vi "capstone1 ver 6.vi"() -> ()   [LabVIEW 2016]
uses:
  <instrlib>/Dynamixel Motor/Public/Motor Operation/Low Level/Baud Setting.ctl
  <vilib>/myRIO/Instrument Drivers/Onboard IO/DIO/typedefs/DIO Reference.ctl
  <vilib>/myRIO/Common/Instrument Driver Framework/Utilities/typedefs/myRIO Generic Hardware Reference.ctl
  <vilib>/myRIO/Common/Instrument Driver Framework/Utilities/typedefs/Hardware Version Enum.ctl
  <vilib>/myRIO/Common/Instrument Driver Framework/Utilities/typedefs/myRIO v1.0 Reference.ctl
  <vilib>/myRIO/Common/Instrument Driver Framework/Utilities/typedefs/Generic FPGA Reference.ctl
  <vilib>/myRIO/Common/Instrument Driver Framework/myRIO v1.0/DIO/typedefs/DIO Channels List.ctl
  <vilib>/myRIO/Common/Instrument Driver Framework/myRIO v1.0/DIO/typedefs/DIO Channels Enum.ctl
  <vilib>/userdefined/High Color/nirio_resource_hc.ctl
  <vilib>/myRIO/Instrument Drivers/Onboard IO/AI/typedefs/AI Reference.ctl
  <vilib>/myRIO/Common/Instrument Driver Framework/myRIO v1.0/AI/typedefs/AI Channels List.ctl
  <vilib>/myRIO/Common/Instrument Driver Framework/myRIO v1.0/AI/typedefs/AI Channels Enum.ctl
  <vilib>/myRIO/Common/Instrument Driver Framework/Utilities/typedefs/Analog Scaling Constants List.ctl
  <vilib>/myRIO/Common/Instrument Driver Framework/Utilities/typedefs/Analog Scaling Constants.ctl
  <vilib>/myRIO/Instrument Drivers/Onboard IO/AO/typedefs/AO Reference.ctl
  <vilib>/myRIO/Common/Instrument Driver Framework/myRIO v1.0/AO/typedefs/AO Channels List.ctl
  <vilib>/myRIO/Common/Instrument Driver Framework/myRIO v1.0/AO/typedefs/AO Channels Enum.ctl
  <vilib>/myRIO/Common/Instrument Driver Framework/Utilities/vis/Is FPGA Ref Available.vi
  <vilib>/myRIO/Common/Instrument Driver Framework/myRIO v1.0/DIO/vis/myRIO v1.1 Open DIO.vi
  <vilib>/myRIO/Instrument Drivers/Onboard IO/DIO/vis/Write.vi
  <vilib>/myRIO/Common/Instrument Driver Framework/myRIO v1.0/AI/vis/myRIO v1.1 Open AI.vi
  <vilib>/myRIO/Instrument Drivers/Onboard IO/AI/vis/Read.vi
  <vilib>/myRIO/Common/Instrument Driver Framework/myRIO v1.0/AO/vis/myRIO v1.1 Open AO.vi
  <vilib>/myRIO/Instrument Drivers/Onboard IO/AO/vis/Write.vi
  <vilib>/myRIO/Common/Instrument Driver Framework/Utilities/vis/Validate Channels.vi
  <vilib>/myRIO/Common/Instrument Driver Framework/myRIO v1.0/DIO/vis/myRIO v1.0 Reserve DIO.vi
  <vilib>/myRIO/Common/Instrument Driver Framework/myRIO v1.0/AI/vis/myRIO v1.0 Reserve AI.vi
  <vilib>/myRIO/Common/Instrument Driver Framework/myRIO v1.0/AO/vis/myRIO v1.0 Reserve AO.vi
  <vilib>/myRIO/Common/Instrument Driver Framework/myRIO v1.0/UART/vis/myRIO v1.0 Close UART.vi
  <vilib>/myRIO/Common/Instrument Driver Framework/myRIO v1.0/Resource Manager/vis/myRIO v1.0 Reserve Channel List.vi
  <vilib>/myRIO/Common/Instrument Driver Framework/myRIO v1.0/DIO/vis/myRIO v1.0 Build MUX Configuration DIO.vi
  <vilib>/myRIO/Common/Instrument Driver Framework/myRIO v1.0/AI/vis/myRIO v1.0 Build MUX Configuration AI.vi
  <vilib>/myRIO/Common/Instrument Driver Framework/myRIO v1.0/AO/vis/myRIO v1.0 Build MUX Configuration AO.vi
  <vilib>/myRIO/Common/Instrument Driver Framework/myRIO v1.0/Resource Manager/vis/myRIO v1.0 Reserve Channel.vi
  <vilib>/myRIO/Common/Instrument Driver Framework/myRIO v1.0/Resource Manager/vis/myRIO v1.0 Unreserve Channel.vi
  <vilib>/myRIO/Common/Instrument Driver Framework/myRIO v1.0/Resource Manager/vis/myRIO v1.0 Create Configuration List.vi
  <vilib>/myRIO/Common/Instrument Driver Framework/myRIO v1.0/Resource Manager/vis/myRIO v1.0 Build Mutex Name.vi
  <vilib>/Utility/VariantDataType/GetNumericInfo.vi
  <vilib>/Utility/error.llb/Error Cluster From Error Code.vi
  <vilib>/myRIO/Common/Instrument Driver Framework/myRIO v1.0/myRIO v1.1 Open.vi
  <vilib>/myRIO/Common/Instrument Driver Framework/Utilities/vis/IO Manager.vi
  <vilib>/myRIO/Common/Instrument Driver Framework/Utilities/vis/Configuration Manager.vi
  <vilib>/myRIO/Common/Instrument Driver Framework/myRIO v1.0/Resource Manager/vis/myRIO v1.0 Configure IO.vi
  <vilib>/myRIO/Common/Instrument Driver Framework/myRIO v1.0/myRIO v1.0 Close.vi
  <vilib>/myRIO/Common/Instrument Driver Framework/myRIO v1.0/DIO/vis/myRIO v1.0 Write DIO.vi
  <vilib>/myRIO/Common/Instrument Driver Framework/myRIO v1.0/AI/vis/myRIO v1.0 Get Scaling Constants AI.vi
  <vilib>/myRIO/Common/Instrument Driver Framework/myRIO v1.0/AI/vis/myRIO v1.0 Read AI.vi
  <vilib>/myRIO/Common/Instrument Driver Framework/myRIO v1.0/AO/vis/myRIO v1.0 Get Scaling Constants AO.vi
  <vilib>/myRIO/Common/Instrument Driver Framework/myRIO v1.0/AO/vis/myRIO v1.0 Write AO.vi
  <vilib>/myRIO/Common/Instrument Driver Framework/Utilities/vis/FPGA Ref Manager.vi
  <vilib>/myRIO/Common/Instrument Driver Framework/myRIO v1.0/myRIO v1.0 Reset FPGA.vi
  <vilib>/myRIO/Common/Instrument Driver Framework/myRIO v1.0/IRQ/vis/myRIO v1.0 IRQ Info FGV.vi
  <vilib>/myRIO/Common/Instrument Driver Framework/myRIO v1.0/IRQ/vis/myRIO v1.0 Timer IRQ Info FGV.vi
  <vilib>/myRIO/Common/Instrument Driver Framework/myRIO v1.0/IRQ/vis/myRIO v1.0 ISR Agent.vi
  <vilib>/myRIO/Express VI/Onboard Devices/LED/LED Express VI.xnode
  <vilib>/myRIO/Instrument Drivers/Onboard IO/DIO/vis/myRIO DIO Open.xnode
  <vilib>/myRIO/Express VI/Onboard IO/AI/AI Express VI.xnode
  <vilib>/myRIO/Instrument Drivers/Onboard IO/AI/vis/myRIO AI Open.xnode
  <vilib>/myRIO/Express VI/Onboard IO/AO/AO Express VI.xnode
  <vilib>/myRIO/Instrument Drivers/Onboard IO/AO/vis/myRIO AO Open.xnode
  <instrlib>/Dynamixel Motor/Dynamixel Motor.lvlib
  <vilib>/myRIO/Instrument Drivers/Onboard IO/DIO/DIO.lvlib
  <vilib>/myRIO/Instrument Drivers/Utilities/Utilities.lvlib
  <vilib>/myRIO/Instrument Drivers/Onboard IO/AO/AO.lvlib
  <vilib>/myRIO/Instrument Drivers/Onboard IO/AI/AI.lvlib
panel:
  out "Load/torque % 3":sgl
  out "Load/torque % 2":sgl
  out "Load/torque %":sgl
  in  "main stop":bool
  out "RT TCP Loop time":u32
  out "motor temp":cluster{"0":sgl, "1":sgl, "2":sgl, "3":sgl}
  out "value":T1
  out "TCP Read data":string
  in  "정지":bool
  out "error out":errorcluster
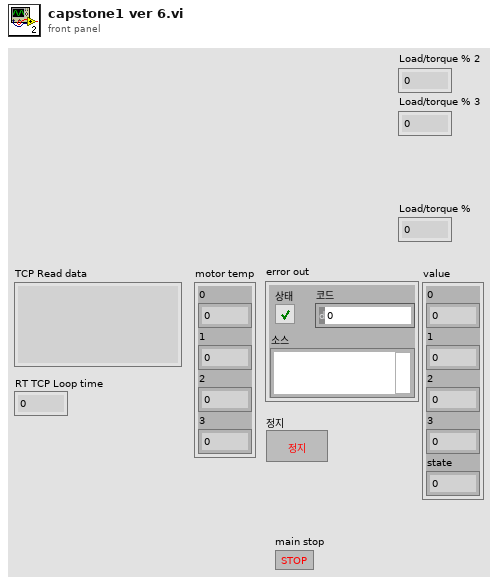
[diagram p1: front panel]
types:
  T1 = cluster{"0":sgl, "1":sgl, "2":sgl, "3":sgl, "state":sgl}
  T2 = typedef "DIO.lvlib/DIO Reference.ctl" = cluster{"myRIO Reference":T3, "DIO Channels List":T7}
  T3 = typedef "myRIO Generic Hardware Reference.ctl" = cluster{"myRIO Model":T4, "myRIO Hardware Reference":T5}
  T4 = typedef "Hardware Version Enum.ctl" = enum16{"Unknown", "myRIO-1900", "myRIO-1950", "roboRIO", "NI ELVIS RIO CM"}
  T5 = typedef "myRIO v1.0 Reference.ctl" = cluster{"Generic FPGA Reference":T6, "Allow multiple opens":bool}
  T6 = typedef "Generic FPGA Reference.ctl" = refnum<k20>
  T7 = typedef "DIO Channels List.ctl" = T8[]
  T8 = typedef "DIO Channels Enum.ctl" = enum16{"Not Connected", "C/DIO0", "C/DIO1", "C/DIO2", "C/DIO3", "C/DIO4", "C/DIO5", "C/DIO6", "C/DIO7", "A/DIO0", "A/DIO1", "A/DIO2", "A/DIO3", "A/DIO4", "A/DIO5", "A/DIO6", "A/DIO7", "A/DIO8", "A/DIO9", "A/DIO10", "A/DIO11", "A/DIO12", "A/DIO13", "A/DIO14", "A/DIO15", "B/DIO0", "B/DIO1", "B/DIO2", "B/DIO3", "B/DIO4", "B/DIO5", "B/DIO6", "B/DIO7", "B/DIO8", "B/DIO9", "B/DIO10", "B/DIO11", "B/DIO12", "B/DIO13", "B/DIO14", "B/DIO15", "LED0", "LED1", "LED2", "LED3", "Button0", "DIO/DIO0", "DIO/DIO1", "DIO/DIO2", "DIO/DIO3", "DIO/DIO4", "DIO/DIO5", "DIO/DIO6", "DIO/DIO7", "DIO/DIO8", "DIO/DIO9", "SPI/CS0", "SPI/CS1", "SPI/CS2", "SPI/CS3", "LED RADIO (Green)", "LED RADIO (Red)", "LED COMM (Green)", "LED COMM (Red)", "LED MODE (Green)", "LED MODE (Red)"}
  T9 = typedef "nirio_resource_hc.ctl" = tag
  T10 = cluster{"0":sgl, "1":sgl, "2":sgl, "3":sgl, "state":i32}
  T11 = typedef "AI.lvlib/AI Reference.ctl" = cluster{"myRIO Reference":T3, "AI Channels List":T12, "AI Scaling Constants List":T14}
  T12 = typedef "AI Channels List.ctl" = T13[]
  T13 = typedef "AI Channels Enum.ctl" = enum16{"Not Connected", "AudioIn/Left", "AudioIn/Right", "C/AI0", "C/AI1", "A/AI0", "A/AI1", "A/AI2", "A/AI3", "B/AI0", "B/AI1", "B/AI2", "B/AI3", "AI/AI0", "AI/AI1", "AI/AI2", "AI/AI3"}
  T14 = typedef "Analog Scaling Constants List.ctl" = T15[]
  T15 = typedef "Analog Scaling Constants.ctl" = cluster{"LSB Weight (Volts)":dbl, "Offset (Volts)":dbl, "Signed?":bool}
  T16 = typedef "AO.lvlib/AO Reference.ctl" = cluster{"myRIO Reference":T3, "AO Channel List":T17, "AO Scaling Constant List":T14}
  T17 = typedef "AO Channels List.ctl" = T18[]
  T18 = typedef "AO Channels Enum.ctl" = enum16{"Not Connected", "AudioOut/Left", "AudioOut/Right", "C/AO0", "C/AO1", "A/AO0", "A/AO1", "B/AO0", "B/AO1"}
  T19 = enum16{"big-endian, network order", "native, host order", "little-endian"}
  T20 = typedef "Dynamixel Motor.lvlib/Baud Setting.ctl" = u8
  T21 = cluster{"Temperature (C)":u8, "Temperature (C)":u8, "Temperature (C)":u8, "Temperature (C)":u8}
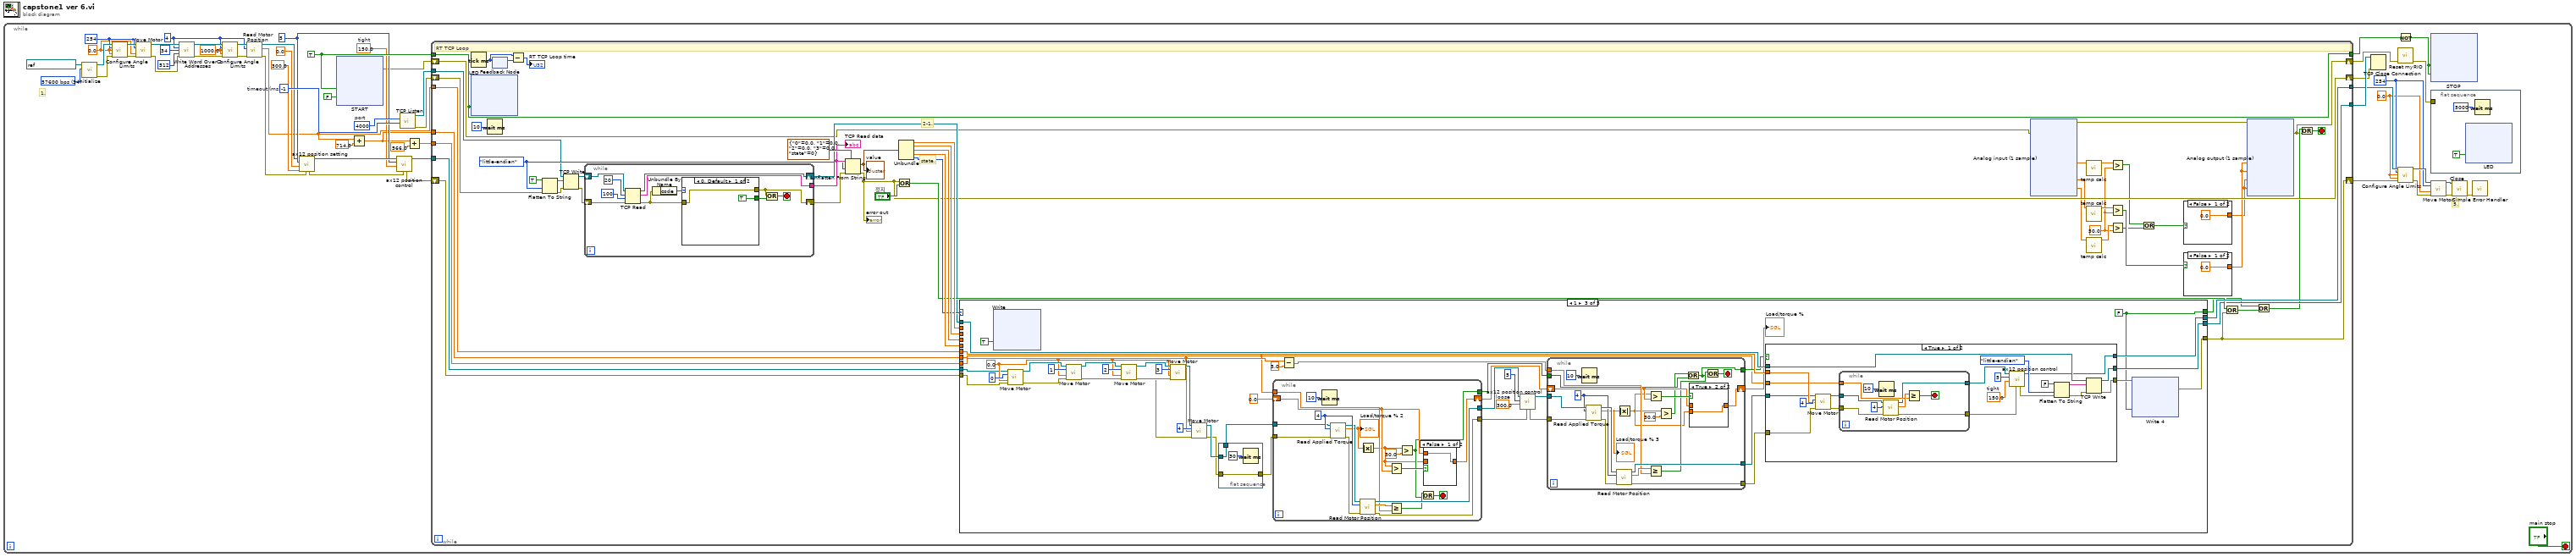
[diagram p0: block diagram]
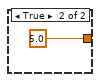
[diagram p2: hidden frame]
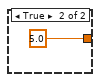
[diagram p3: hidden frame]
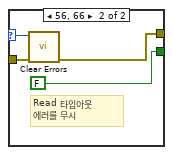
[diagram p4: hidden frame]
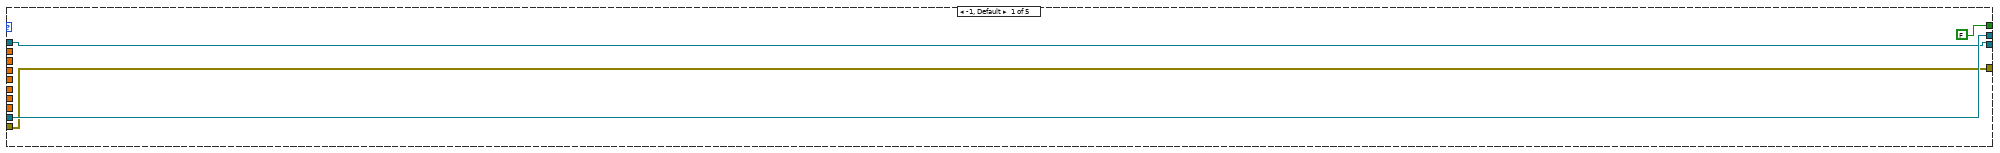
[diagram p5: hidden frame]
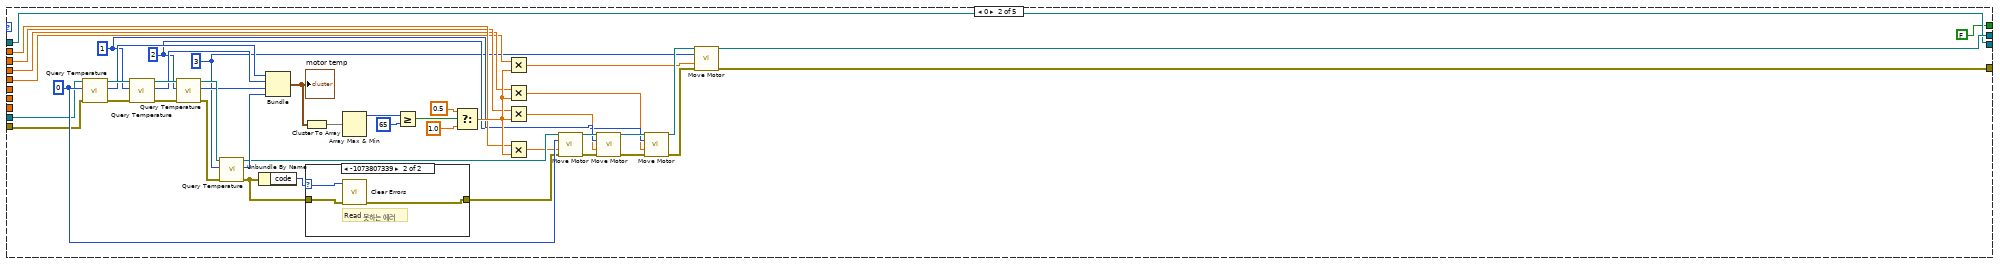
[diagram p6: hidden frame]
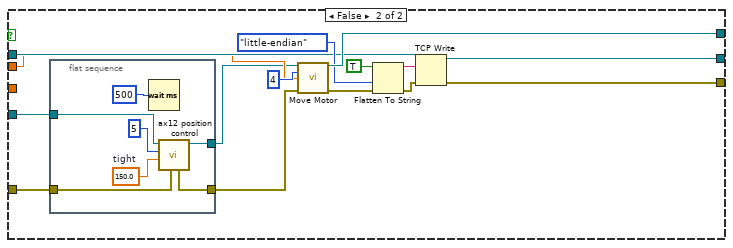
[diagram p8: hidden frame]
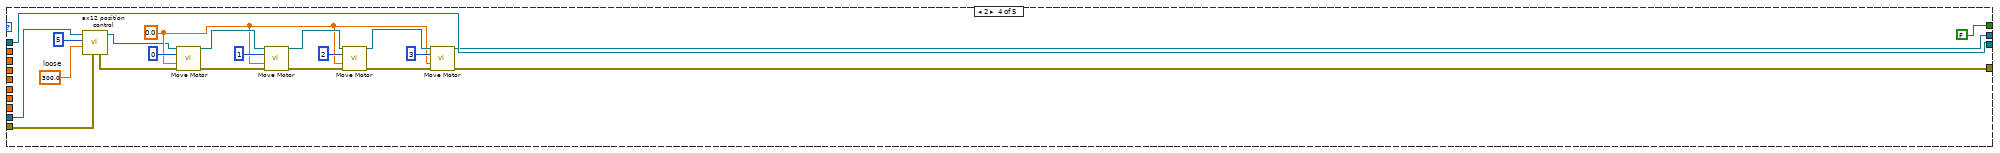
[diagram p11: hidden frame]
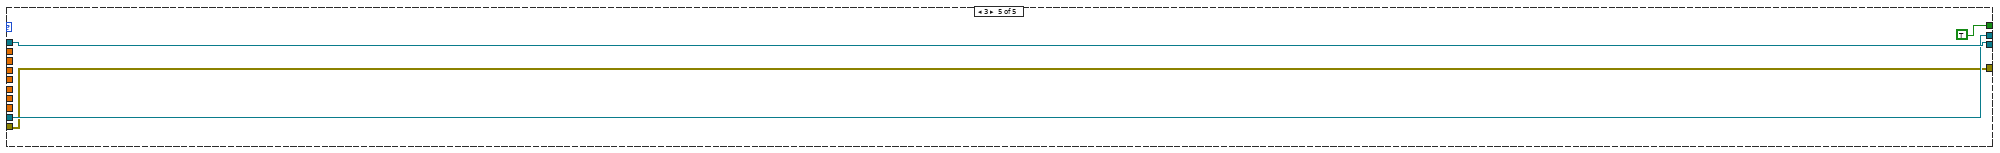
[diagram p12: hidden frame]
diagram:
  n1 = while {
    stop <- "main stop" stop-if-true
    w36 = 1000.0 ("Clockwise Angle Limit (0 deg)")
    w1 = 4
    w29 = 150.0  # tight
    w28 = 5
    w51 = T20 34 items=["1,000,000 bps"=1, "500,000 bps"=3, "400,000 bps"=4, "250,000 bps"=7, "200,000 bps"=9, "115200 bps"=16, "57600 bps"=34, "19200 bps"=103, "9600 bps"=207] ("Baud rate (57600 bps)")
    w41 = TRUE
    w22 = 0.0 ("Goal Speed (RPM)")
    w23 = u8 254 ("Motor ID (0)")
    w43 = u8 254 ("Motor ID (0)")
    w42 = 0.0 ("Clockwise Angle Limit (0 deg)")
    w55 = u16 4000  # port
    w56 = -1  # timeout (ms)
    # "5."
    # "1."
    n2 = call <instrlib>:"Initialize.vi"("Baud rate (57600 bps)"=w51, "VISA resource name"=refnum<visa-resource-name> "ASRL3::INSTR") -> ("error out"=w47:errorcluster, "VISA resource name out"=w46:refnum<visa-resource-name>)  [unwired: 8 in]
    n3 = call <instrlib>:"Configure Angle Limits.vi"("VISA resource name"=w46, "Motor ID (0)"=w43, "Clockwise Angle Limit (0 deg)"=w42, "Counter-Clockwise Angle Limit (300 deg)"=w42, "error in (no error)"=w47) -> ("VISA resource name out"=w45:refnum<visa-resource-name>, "error out"=w44:errorcluster)  [unwired: 9 in]
    n4 = call <instrlib>:"Move Motor.vi"("VISA resource name"=w45, "Motor ID (0)"=w43, "Goal Speed (RPM)"=w42, "error in (no error)"=w44) -> ("VISA resource name out"=w5:refnum<visa-resource-name>, "error out"=w4:errorcluster)  [unwired: 10 in]
    n5 = call <instrlib>:"Write Word Over 2 Addresses.vi"("VISA resource name"=w5, "Motor ID (0)"=w1, "Address number (0)"=u8 34, "Parameter (0)"=u16 512, "error in (no error)"=w4) -> ("VISA resource name out"=w2:refnum<visa-resource-name>, "error out"=w3:errorcluster)  [unwired: 9 in]
    n6 = call <instrlib>:"Configure Angle Limits.vi"("VISA resource name"=w2, "Motor ID (0)"=w1, "Clockwise Angle Limit (0 deg)"=w36, "Counter-Clockwise Angle Limit (300 deg)"=w36, "error in (no error)"=w3) -> ("VISA resource name out"=w21:refnum<visa-resource-name>, "error out"=w18:errorcluster)  [unwired: 9 in]
    n7 = call <instrlib>:"Read Motor Position.vi"("error in (no error)"=w18, "Motor ID (0)"=w1, "VISA resource name"=w21) -> ("error out"=w19:errorcluster, "Position (deg)"=w13:dbl, "VISA resource name out"=w20:refnum<visa-resource-name>)  [unwired: 6 in]
    n8 = call "ax12 position setting.vi"("error in (no error)"=w19, "Counter-Clockwise Angle Limit (300 deg)"=300.0 ("Clockwise Angle Limit (0 deg)"), "Clockwise Angle Limit (0 deg)"=0.0, "Motor ID (0)"=w28, "VISA resource name"=w20) -> ("VISA resource name out"=w33:refnum<visa-resource-name>, "error out"=w30:errorcluster)  [unwired: 5 in]
    n9 = xnode "START"("LED0"=w41, "LED3"=FALSE) -> ("error out"=w9:errorcluster)  [unwired: 1 in]
    n10 = Add(x=w13, y=714.0) -> (x+y=w14:dbl)
    n11 = call "ax12 position control.vi"("error in (no error)"=w30, "Goal Position (180 deg)"=w29, "Motor ID (0)"=w28, "VISA resource name"=w33) -> ("VISA resource name out"=w32:refnum<visa-resource-name>, "error out"=w31:errorcluster)  [unwired: 6 in]
    n12 = call <vilib>:"TCP Listen.vi"("timeout ms (wait forever: -1)"=w56, "port"=w55) -> ("error out"=w52:errorcluster, "connection ID"=w38:refnum<k5>)  [unwired: 5 in, 3 out]
    n13 = Add(x=w14, y=566.0) -> (x+y=w15:dbl)
    n14 = while {
      tunnel: w38 -> [w190]
      tunnel: [w198] -> w54
      shift-right: [w184] -> w53
      shift-left: w52 -> [w187]
      shift-right: [w207] -> w27
      shift-left: w31 -> [w206]
      tunnel: w41 -> [w215]
      tunnel: [w215] -> w49
      tunnel: [w208] -> w25
      tunnel: w32 -> [w200]
      tunnel: w15 -> [w197]
      tunnel: w14 -> [w196]
      tunnel: w13 -> [w195]
      shift-right: [w175] -> w8
      shift-left: w9 -> [w178]
      stop <- w174 stop-if-true
      w180 = 50.0 ("y")
      w191 = T19."little-endian" ("byte order (0:big-endian, network order)")
      # "state."
      # "2-1."
      # "RT TCP Loop"
      n15 = Tick Count (ms)() -> (millisecond timer value=w203:u32)
      n16 = xnode "LED"("LED1"=w215) -> ()  [unwired: 1 in, 1 out]
      n17 = Wait (ms)(milliseconds to wait=u32 10 ("대기 시간 (ms)")) -> ()  [unwired: 1 out]
      n18 = feedback #1() -> (w204:u32)  [unwired: 1 in]
      n19 = feedback-in #1(w203) -> ()
      n20 = Subtract(x=w203, y=w204) -> (x-y=→"RT TCP Loop time":u32)
      n21 = Flatten To String(anything=TRUE, byte order (0:big-endian, network order)=w191, error in (no error)=w187) -> (data string=w194:string, error out=w193:errorcluster)  [unwired: 1 in, 1 out]
      n22 = TCP Write(connection ID=w190, data in=w194, error in (no error)=w193) -> (connection ID out=w189:refnum<k5>, error out=w188:errorcluster)  [unwired: 1 in, 1 out]
      n23 = while {
        tunnel: [w312] -> w217
        shift-right: [w311] -> w199
        shift-left: w189 -> [w310]
        shift-right: [w306] -> w216
        shift-left: w188 -> [w309]
        stop <- w304 stop-if-true
        n24 = TCP Read(connection ID=w310, bytes to read=20 ("읽을 바이트"), error in (no error)=w309, 9:100 ("타임아웃 ms (25000)")) -> (connection ID out=w311:refnum<k5>, data out=w312:string, error out=w307:errorcluster)  [unwired: 1 in]
        n25 = Unbundle By Name(w307) -> ("code"=w308:i32)
        n26 = case shown="0, Default" w308 {
          selector: w308 -> [_ w319]
          tunnel: [w316 w318] -> w306
          tunnel: w307 -> [w316 w320]
          tunnel: [TRUE FALSE] -> w305
          frame 0, Default {
          }
          frame 56, 66 {
            # "Read 타임아웃\n에러를 무시"
            n27 = call <vilib>:"Clear Errors.vi"("error in (no error)"=w320, "specific error code to clear (0: all)"=w319) -> ("error out"=w318:errorcluster)  [unwired: 4 in, 1 out]
          }
        }
        n28 = Or(x=w306, y=w305) -> (x .or. y?=w304:bool)
      }
      "TCP Read data" <- w217
      n29 = Unflatten From String(type=T10 {"0"=0.0, "1"=0.0, "2"=0.0, "3"=0.0, "state"=0}, binary string=w217, byte order (0:big-endian, network order)=w191, error in (no error)=w216) -> (value=w214:T10, error out=w184:errorcluster)  [unwired: 1 in, 1 out]
      "error out" <- w184
      "value" <- w214
      n30 = Or(x=w184, y="정지") -> (x .or. y?=w205:bool)
      n31 = Unbundle(w214) -> ("0"=w213:sgl, "1"=w211:sgl, "2"=w212:sgl, "3"=w210:sgl, "state"=w209:i32)
      n32 = case shown="1" w209 {
        tunnel: w213 -> [_ w354 _ _ _]
        tunnel: w211 -> [_ w353 _ _ _]
        tunnel: w212 -> [_ w352 _ _ _]
        tunnel: w210 -> [_ w351 _ _ _]
        tunnel: [w324 w336 w396 w590 w611] -> w208
        tunnel: [w323 w337 w392 w589 w610] -> w207
        tunnel: w206 -> [w323 w334 w408 w595 w610]
        tunnel: w200 -> [w324 w327 w406 w594 w611]
        tunnel: w199 -> [w322 w326 w394 w597 w612]
        tunnel: [w322 w326 w395 w597 w612] -> w198
        tunnel: w197 -> [_ _ w390 _ _]
        tunnel: w196 -> [_ _ w379 _ _]
        tunnel: w195 -> [_ _ w391 _ _]
        tunnel: [FALSE FALSE w385 FALSE TRUE] -> w186
        frame -1, Default {
        }
        frame 0 {
          w338 = 3
          w339 = 2
          w340 = 1
          w335 = 0
          n33 = call <instrlib>:"Query Temperature.vi"("error in"=w334, "Motor ID (0)"=w335, "VISA resource name"=w327) -> ("error out"=w361:errorcluster, "Temperature (C)"=w350:u8, "VISA resource name out"=w364:refnum<visa-resource-name>)  [unwired: 6 in]
          n34 = call <instrlib>:"Query Temperature.vi"("error in"=w361, "Motor ID (0)"=w340, "VISA resource name"=w364) -> ("error out"=w360:errorcluster, "Temperature (C)"=w349:u8, "VISA resource name out"=w363:refnum<visa-resource-name>)  [unwired: 6 in]
          n35 = call <instrlib>:"Query Temperature.vi"("error in"=w360, "Motor ID (0)"=w339, "VISA resource name"=w363) -> ("error out"=w359:errorcluster, "Temperature (C)"=w348:u8, "VISA resource name out"=w362:refnum<visa-resource-name>)  [unwired: 6 in]
          n36 = call <instrlib>:"Query Temperature.vi"("error in"=w359, "Motor ID (0)"=w338, "VISA resource name"=w362) -> ("error out"=w341:errorcluster, "Temperature (C)"=w347:u8, "VISA resource name out"=w333:refnum<visa-resource-name>)  [unwired: 6 in]
          n37 = Unbundle By Name(w341) -> ("code"=w342:i32)
          n38 = Bundle("Temperature (C)"=w350, "Temperature (C)"=w349, "Temperature (C)"=w348, "Temperature (C)"=w347) -> (w344:T21)  [unwired: 1 in]
          "motor temp" <- w344
          n39 = Cluster To Array(cluster=w344) -> (array=w346:u8[])
          n40 = case shown="-1073807339" w342 {
            selector: w342 -> [_ w373]
            tunnel: [w371 w372] -> w332
            tunnel: w341 -> [w371 w374]
            frame 0, Default {
            }
            frame -1073807339 {
              # "Read 못하는 에러"
              n41 = call <vilib>:"Clear Errors.vi"("error in (no error)"=w374, "specific error code to clear (0: all)"=w373) -> ("error out"=w372:errorcluster)  [unwired: 4 in, 1 out]
            }
          }
          n42 = Array Max & Min(array=w346) -> (max value=w345:u8)  [unwired: 3 out]
          n43 = Greater Or Equal?(x=w345, y=65) -> (x >= y?=w343:bool)
          n44 = Select(t=0.5, s=w343, f=1.0) -> (s? t:f=w355:dbl)
          n45 = Multiply(x=w351, y=w355) -> (x*y=w328:dbl)
          n46 = Multiply(x=w352, y=w355) -> (x*y=w329:dbl)
          n47 = Multiply(x=w353, y=w355) -> (x*y=w330:dbl)
          n48 = Multiply(x=w354, y=w355) -> (x*y=w331:dbl)
          n49 = call <instrlib>:"Move Motor.vi"("VISA resource name"=w333, "Motor ID (0)"=w335, "Goal Speed (RPM)"=w331, "error in (no error)"=w332) -> ("VISA resource name out"=w365:refnum<visa-resource-name>, "error out"=w366:errorcluster)  [unwired: 10 in]
          n50 = call <instrlib>:"Move Motor.vi"("VISA resource name"=w365, "Motor ID (0)"=w340, "Goal Speed (RPM)"=w330, "error in (no error)"=w366) -> ("VISA resource name out"=w367:refnum<visa-resource-name>, "error out"=w369:errorcluster)  [unwired: 10 in]
          n51 = call <instrlib>:"Move Motor.vi"("VISA resource name"=w367, "Motor ID (0)"=w339, "Goal Speed (RPM)"=w329, "error in (no error)"=w369) -> ("VISA resource name out"=w368:refnum<visa-resource-name>, "error out"=w370:errorcluster)  [unwired: 10 in]
          n52 = call <instrlib>:"Move Motor.vi"("VISA resource name"=w368, "Motor ID (0)"=w338, "Goal Speed (RPM)"=w328, "error in (no error)"=w370) -> ("VISA resource name out"=w336:refnum<visa-resource-name>, "error out"=w337:errorcluster)  [unwired: 10 in]
        }
        frame 1 {
          w385 = FALSE ("notification")
          w400 = 300.0  # loose
          w409 = 0.0
          n53 = xnode "Write"("LED2"=TRUE) -> ()  [unwired: 1 in, 1 out]
          n54 = call <instrlib>:"Move Motor.vi"("VISA resource name"=w406, "Motor ID (0)"=0, "Goal Speed (RPM)"=w409, "error in (no error)"=w408) -> ("VISA resource name out"=w410:refnum<visa-resource-name>, "error out"=w411:errorcluster)  [unwired: 10 in]
          n55 = call <instrlib>:"Move Motor.vi"("VISA resource name"=w410, "Motor ID (0)"=1, "Goal Speed (RPM)"=w409, "error in (no error)"=w411) -> ("VISA resource name out"=w412:refnum<visa-resource-name>, "error out"=w414:errorcluster)  [unwired: 10 in]
          n56 = call <instrlib>:"Move Motor.vi"("VISA resource name"=w412, "Motor ID (0)"=2, "Goal Speed (RPM)"=w409, "error in (no error)"=w414) -> ("VISA resource name out"=w413:refnum<visa-resource-name>, "error out"=w415:errorcluster)  [unwired: 10 in]
          n57 = call <instrlib>:"Move Motor.vi"("VISA resource name"=w413, "Motor ID (0)"=3, "Goal Speed (RPM)"=w409, "error in (no error)"=w415) -> ("VISA resource name out"=w404:refnum<visa-resource-name>, "error out"=w405:errorcluster)  [unwired: 10 in]
          n58 = call <instrlib>:"Move Motor.vi"("VISA resource name"=w404, "Motor ID (0)"=4, "Goal Position (180 deg)"=w390, "error in (no error)"=w405) -> ("VISA resource name out"=w378:refnum<visa-resource-name>, "error out"=w377:errorcluster)  [unwired: 10 in]
          n59 = flat-sequence {
            tunnel: w378 -> [w421]
            tunnel: w377 -> [w420]
            tunnel: [w421] -> w376
            tunnel: [w420] -> w375
            frame #0 {
              n60 = Wait (ms)(milliseconds to wait=u32 30 ("대기 시간 (ms)")) -> ()  [unwired: 1 out]
            }
          }
          n61 = while {
            tunnel: w376 -> [w542]
            tunnel: w375 -> [w545]
            tunnel: [w548] -> w402
            tunnel: [w547] -> w401
            tunnel: w379 -> [w546]
            shift-right: [w538] -> w383
            shift-left: sgl 0.0 ("Load/torque %") -> [w539]
            tunnel: [w534] -> w381
            stop <- w535 stop-if-true
            w543 = 4
            n62 = Wait (ms)(milliseconds to wait=u32 10 ("대기 시간 (ms)")) -> ()  [unwired: 1 out]
            n63 = call <instrlib>:"Read Applied Torque.vi"("error in (no error)"=w545, "Motor ID (0)"=w543, "VISA resource name"=w542) -> ("error out"=w544:errorcluster, "Load/torque %"=w533:sgl, "VISA resource name out"=w541:refnum<visa-resource-name>)  [unwired: 6 in]
            "Load/torque % 2" <- w533
            n64 = call <instrlib>:"Read Motor Position.vi"("error in (no error)"=w544, "Motor ID (0)"=w543, "VISA resource name"=w541) -> ("error out"=w547:errorcluster, "Position (deg)"=w549:dbl, "VISA resource name out"=w548:refnum<visa-resource-name>)  [unwired: 6 in]
            n65 = Absolute Value(x=w533) -> (abs(x)=w532:sgl)
            n66 = Greater?(x=w532, y=w539) -> (0:w540:bool)
            n67 = Greater Or Equal?(x=w549, y=w546) -> (x >= y?=w536:bool)
            n68 = Greater?(x=w532, y=sgl 30.0) -> (0:w534:bool)
            n69 = Or(x=w536, y=w534) -> (x .or. y?=w535:bool)
            n70 = case shown="False" w540 {
              tunnel: [w551 w552] -> w538
              tunnel: w532 -> [_ w552]
              tunnel: w539 -> [w551 _]
              frame False {
              }
              frame True {
              }
            }
          }
          n71 = Subtract(x=w390, y=3.0) -> (x-y=w388:dbl)
          n72 = call "ax12 position control.vi"("error in (no error)"=w401, "Goal Position (180 deg)"=w400, "Motor ID (0)"=u8 5, "VISA resource name"=w402) -> ("VISA resource name out"=w398:refnum<visa-resource-name>, "error out"=w397:errorcluster)  [unwired: 6 in]
          n73 = while {
            tunnel: w398 -> [w524]
            tunnel: w397 -> [w523]
            tunnel: [w527] -> w387
            tunnel: [w526] -> w386
            tunnel: w388 -> [w525]
            shift-right: [w517] -> w382
            shift-left: w383 -> [w518]
            tunnel: w381 -> [w514]
            tunnel: [w511] -> w380
            stop <- w513 stop-if-true
            w520 = 4
            n74 = Wait (ms)(milliseconds to wait=u32 10 ("대기 시간 (ms)")) -> ()  [unwired: 1 out]
            n75 = call <instrlib>:"Read Applied Torque.vi"("error in (no error)"=w523, "Motor ID (0)"=w520, "VISA resource name"=w524) -> ("error out"=w522:errorcluster, "Load/torque %"=w510:sgl, "VISA resource name out"=w521:refnum<visa-resource-name>)  [unwired: 6 in]
            "Load/torque % 3" <- w510
            n76 = call <instrlib>:"Read Motor Position.vi"("error in (no error)"=w522, "Motor ID (0)"=w520, "VISA resource name"=w521) -> ("error out"=w526:errorcluster, "Position (deg)"=w528:dbl, "VISA resource name out"=w527:refnum<visa-resource-name>)  [unwired: 6 in]
            n77 = Absolute Value(x=w510) -> (abs(x)=w509:sgl)
            n78 = Greater?(x=w509, y=w518) -> (0:w519:bool)
            n79 = Greater Or Equal?(x=w528, y=w525) -> (x >= y?=w515:bool)
            n80 = Greater?(x=w509, y=sgl 30.0) -> (0:w512:bool)
            n81 = Or(x=w512, y=w514) -> (x .or. y?=w511:bool)
            n82 = case shown="True" w519 {
              tunnel: [w530 w531] -> w517
              tunnel: w509 -> [_ w531]
              tunnel: w518 -> [w530 _]
              frame False {
              }
              frame True {
              }
            }
            n83 = Or(x=w515, y=w511) -> (x .or. y?=w513:bool)
          }
          "Load/torque %" <- w382
          n84 = case shown="True" w380 {
            tunnel: [w425 w465] -> w396
            tunnel: [w438 w461] -> w395
            tunnel: w394 -> [w437 w460]
            tunnel: [w436 w458] -> w393
            tunnel: w391 -> [w435 w457]
            tunnel: w387 -> [w433 w456]
            tunnel: w386 -> [w434 w455]
            tunnel: w379 -> [w430 _]
            frame True {
              w428 = 150.0  # tight
              n85 = call <instrlib>:"Move Motor.vi"("VISA resource name"=w433, "Motor ID (0)"=4, "Goal Position (180 deg)"=w435, "error in (no error)"=w434) -> ("VISA resource name out"=w432:refnum<visa-resource-name>, "error out"=w431:errorcluster)  [unwired: 10 in]
              n86 = while {
                tunnel: w432 -> [w451]
                tunnel: w431 -> [w450]
                tunnel: w430 -> [w446]
                tunnel: [w444] -> w427
                tunnel: [w443] -> w426
                stop <- w445 stop-if-true
                n87 = Wait (ms)(milliseconds to wait=u32 10 ("대기 시간 (ms)")) -> ()  [unwired: 1 out]
                n88 = call <instrlib>:"Read Motor Position.vi"("error in (no error)"=w450, "Motor ID (0)"=4, "VISA resource name"=w451) -> ("error out"=w443:errorcluster, "Position (deg)"=w447:dbl, "VISA resource name out"=w444:refnum<visa-resource-name>)  [unwired: 6 in]
                n89 = Greater Or Equal?(x=w447, y=w446) -> (x >= y?=w445:bool)
              }
              n90 = call "ax12 position control.vi"("error in (no error)"=w426, "Goal Position (180 deg)"=w428, "Motor ID (0)"=u8 5, "VISA resource name"=w427) -> ("VISA resource name out"=w425:refnum<visa-resource-name>, "error out"=w424:errorcluster)  [unwired: 6 in]
              n91 = Flatten To String(anything=FALSE, byte order (0:big-endian, network order)=T19."little-endian", error in (no error)=w424) -> (data string=w440:string, error out=w439:errorcluster)  [unwired: 1 in, 1 out]
              n92 = TCP Write(connection ID=w437, data in=w440, error in (no error)=w439) -> (connection ID out=w438:refnum<k5>, error out=w436:errorcluster)  [unwired: 1 in, 1 out]
            }
            frame False {
              n93 = flat-sequence {
                tunnel: w456 -> [w470]
                tunnel: w455 -> [w469]
                tunnel: [w468] -> w454
                tunnel: [w467] -> w453
                frame #0 {
                  w471 = 150.0  # tight
                  n94 = Wait (ms)(milliseconds to wait=u32 500) -> ()  [unwired: 1 out]
                  n95 = call "ax12 position control.vi"("error in (no error)"=w469, "Goal Position (180 deg)"=w471, "Motor ID (0)"=u8 5, "VISA resource name"=w470) -> ("VISA resource name out"=w468:refnum<visa-resource-name>, "error out"=w467:errorcluster)  [unwired: 6 in]
                }
              }
              n96 = call <instrlib>:"Move Motor.vi"("VISA resource name"=w454, "Motor ID (0)"=4, "Goal Position (180 deg)"=w457, "error in (no error)"=w453) -> ("VISA resource name out"=w465:refnum<visa-resource-name>, "error out"=w459:errorcluster)  [unwired: 10 in]
              n97 = Flatten To String(anything=TRUE, byte order (0:big-endian, network order)=T19."little-endian", error in (no error)=w459) -> (data string=w463:string, error out=w462:errorcluster)  [unwired: 1 in, 1 out]
              n98 = TCP Write(connection ID=w460, data in=w463, error in (no error)=w462) -> (connection ID out=w461:refnum<k5>, error out=w458:errorcluster)  [unwired: 1 in, 1 out]
            }
          }
          n99 = xnode "Write 4"("LED2"=w385, "error in (no error)"=w393) -> ("error out"=w392:errorcluster)
        }
        frame 2 {
          w591 = 300.0  # loose
          w598 = 0.0
          n100 = call "ax12 position control.vi"("error in (no error)"=w595, "Goal Position (180 deg)"=w591, "Motor ID (0)"=5, "VISA resource name"=w594) -> ("VISA resource name out"=w593:refnum<visa-resource-name>, "error out"=w596:errorcluster)  [unwired: 6 in]
          n101 = call <instrlib>:"Move Motor.vi"("VISA resource name"=w593, "Motor ID (0)"=0, "Goal Speed (RPM)"=w598, "error in (no error)"=w596) -> ("VISA resource name out"=w608:refnum<visa-resource-name>, "error out"=w607:errorcluster)  [unwired: 10 in]
          n102 = call <instrlib>:"Move Motor.vi"("VISA resource name"=w608, "Motor ID (0)"=1, "Goal Speed (RPM)"=w598, "error in (no error)"=w607) -> ("VISA resource name out"=w606:refnum<visa-resource-name>, "error out"=w604:errorcluster)  [unwired: 10 in]
          n103 = call <instrlib>:"Move Motor.vi"("VISA resource name"=w606, "Motor ID (0)"=2, "Goal Speed (RPM)"=w598, "error in (no error)"=w604) -> ("VISA resource name out"=w605:refnum<visa-resource-name>, "error out"=w603:errorcluster)  [unwired: 10 in]
          n104 = call <instrlib>:"Move Motor.vi"("VISA resource name"=w605, "Motor ID (0)"=3, "Goal Speed (RPM)"=w598, "error in (no error)"=w603) -> ("VISA resource name out"=w590:refnum<visa-resource-name>, "error out"=w589:errorcluster)  [unwired: 10 in]
        }
        frame 3 {
        }
      }
      n105 = xnode "Analog input (1 sample)"("error in (no error)"=w178) -> ("Myrio (A/AI0 (Pin 3))"=w173:dbl, "Converter (B/AI0 (Pin 3))"=w172:dbl, "NUC (B/AI1 (Pin 5))"=w171:dbl, "error out"=w177:errorcluster)  [unwired: 1 out]
      n106 = call "temp calc.vi"("Numeric"=w173) -> ("x/y"=w183:dbl)  [unwired: 10 in]
      n107 = call "temp calc.vi"("Numeric"=w172) -> ("x/y"=w182:dbl)  [unwired: 10 in]
      n108 = call "temp calc.vi"("Numeric"=w171) -> ("x/y"=w181:dbl)  [unwired: 10 in]
      n109 = Greater?(x=w183, y=w180) -> (0:w169:bool)
      n110 = Greater?(x=w182, y=w180) -> (0:w179:bool)
      n111 = Greater?(x=w181, y=w180) -> (0:w168:bool)
      n112 = Or(x=w169, y=w168) -> (x .or. y?=w167:bool)
      n113 = case shown="False" w167 {
        tunnel: [0.0 5.0] -> w166
        frame False {
        }
        frame True {
        }
      }
      n114 = case shown="False" w179 {
        tunnel: [0.0 5.0] -> w170
        frame False {
        }
        frame True {
        }
      }
      n115 = Or(x=w205, y=w207) -> (x .or. y?=w185:bool)
      n116 = xnode "Analog output (1 sample)"("A/AO0 (Pin 2)"=w170, "A/AO1 (Pin 4)"=w170, "B/AO0 (Pin 2)"=w166, "B/AO1 (Pin 4)"=w166, "error in (no error)"=w177) -> ("error out"=w175:errorcluster)
      n117 = Or(x=w186, y=w185) -> (x .or. y?=w176:bool)
      n118 = Or(x=w176, y=w175) -> (x .or. y?=w174:bool)
    }
    n119 = TCP Close Connection(connection ID=w54, error in (no error)=w53) -> ()  [unwired: 3 out]
    n120 = Not(x=w49) -> (.not. x?=w48:bool)
    n121 = call <vilib>:"Reset myRIO.vi"("error in (no error)"=w8) -> ("error out"=w12:errorcluster)  [unwired: 10 in]
    n122 = call <instrlib>:"Configure Angle Limits.vi"("VISA resource name"=w25, "Motor ID (0)"=w23, "Clockwise Angle Limit (0 deg)"=w22, "Counter-Clockwise Angle Limit (300 deg)"=w22, "error in (no error)"=w27) -> ("VISA resource name out"=w24:refnum<visa-resource-name>, "error out"=w26:errorcluster)  [unwired: 9 in]
    n123 = xnode "STOP"("LED0"=w48, "LED1"=w48) -> ()  [unwired: 1 in, 1 out]
    n124 = flat-sequence {
      tunnel: w12 -> [_]
      frame #0 {
        n125 = xnode "LED"("LED3"=TRUE) -> ()  [unwired: 1 in, 1 out]
        n126 = Wait (ms)(milliseconds to wait=5000) -> ()  [unwired: 1 out]
      }
    }
    n127 = call <instrlib>:"Move Motor.vi"("VISA resource name"=w24, "Motor ID (0)"=w23, "Goal Speed (RPM)"=w22, "error in (no error)"=w26) -> ("VISA resource name out"=w40:refnum<visa-resource-name>, "error out"=w39:errorcluster)  [unwired: 10 in]
    n128 = call <instrlib>:"Close.vi"("error in (no error)"=w39, "VISA resource name"=w40) -> ("error out"=w37:errorcluster)  [unwired: 9 in]
    n129 = call <vilib>:"Simple Error Handler.vi"("error in (no error)"=w37) -> ()  [unwired: 4 in, 5 out]
  }
